vi "Simple Reader.vi"(8 "error in (no error)":errorcluster, 11 "Ocean Optics Driver in":refnum<class "Ocean Optics Driver.lvclass">) -> (0 "error out":errorcluster, 2 "Signals":dbl[](array[numeric]), 3 "Ocean Optics Driver out":refnum<class "Ocean Optics Driver.lvclass">)   [LabVIEW 2016, in "Ocean Optics Driver.lvclass"]
uses:
  Ocean Optics Driver.lvclass
  C:/github/NHMFL_Core/Libraries/Instruments/Instrument Driver/Instrument Driver.lvclass
  Ocean Optics Driver.lvclass/Ocean Optics Driver.ctl
  Instrument Driver/Instrument Driver.lvclass/Instrument Driver.ctl
  Instrument Driver/Write Channel names.vi
  Instrument Driver/Write Channel units.vi
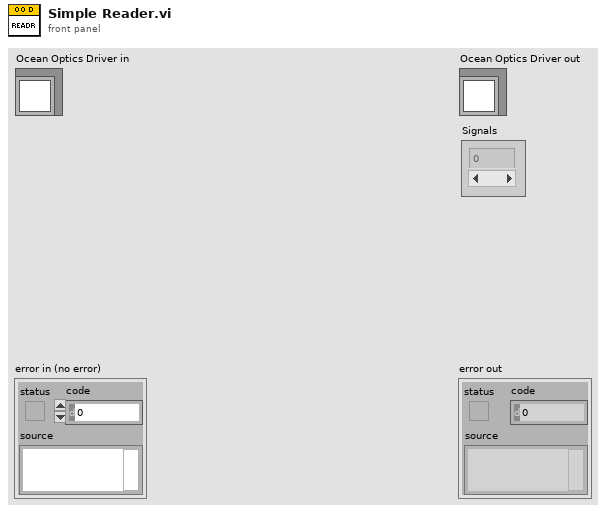
[diagram p1: front panel]
types:
  T1 = typedef "Peak Parameters.ctl" = cluster{"Amplitude":dbl, "Center":dbl, "Width":dbl}
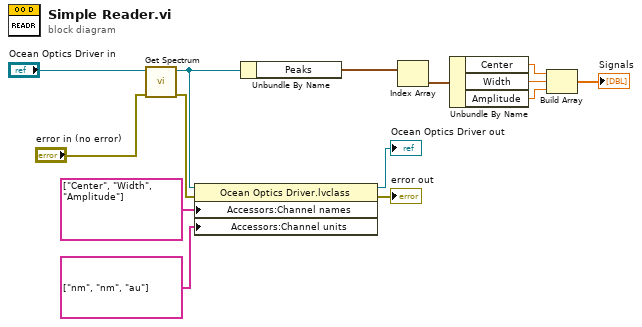
[diagram p0: block diagram]
diagram:
  n1 = call-dynamic "Get Spectrum.vi"("error in (no error)"="error in (no error)", "Ocean Optics Driver in"="Ocean Optics Driver in") -> ("error out"=w1:errorcluster, "Ocean Optics Driver out"=w8:refnum<class "Ocean Optics Driver.lvclass">)  [unwired: 7 in, 1 out]
  n2 = property class="Ocean Optics Driver.lvclass"(reference=w8, error in=w1, "Accessors:Channel names"=string[] ["Center", "Width", "Amplitude"] ("Channel names"), "Accessors:Channel units"=string[] ["nm", "nm", "au"] ("Channel names")) -> (reference out=→"Ocean Optics Driver out":refnum<class "Ocean Optics Driver.lvclass">, error out=→"error out":errorcluster)
  n3 = Unbundle By Name(w8) -> ("Peaks"=w12:T1[])
  n4 = Index Array(array=w12) -> (element=w11:T1)  [unwired: 1 in]
  n5 = Unbundle By Name(w11) -> ("Center"=w10:dbl, "Width"=w7:dbl, "Amplitude"=w6:dbl)
  n6 = Build Array(w10, w7, w6) -> (→"Signals":dbl[])
